vi "LowPressureVerification.vi"(8 "error in":errorcluster, 11 "S1 in":refnum<class "S4.lvclass">) -> (0 "error out":errorcluster, 3 "S1 out":refnum<class "S4.lvclass">)   [LabVIEW 2018, in "S4.lvclass"]
uses:
  S4.lvclass
  S4.lvclass/S4.ctl
  Public Controls/Outputs.ctl
  Public Controls/ReportHeader.ctl
  IO/IO.lvclass
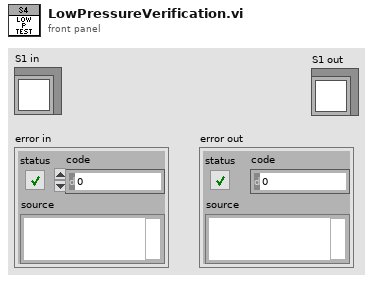
[diagram p1: front panel]
types:
  T1 = typedef "S4.lvclass/Outputs.ctl" = cluster{"LO P":bool, "HI P":bool, "Z3Vent":bool, "V2 Vent":bool, "IsLidLocked":bool}
  T2 = typedef "S4.lvclass/ReportHeader.ctl" = string
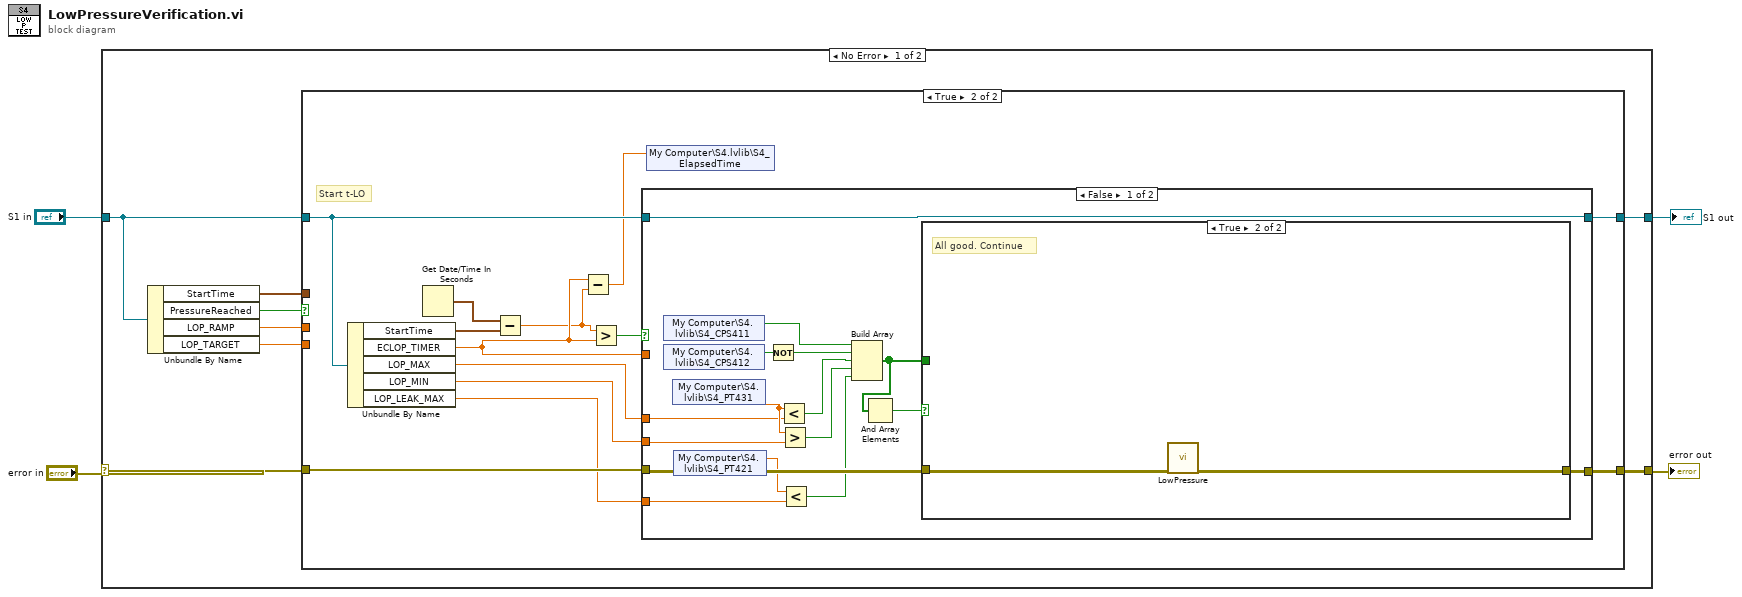
[diagram p0: block diagram]
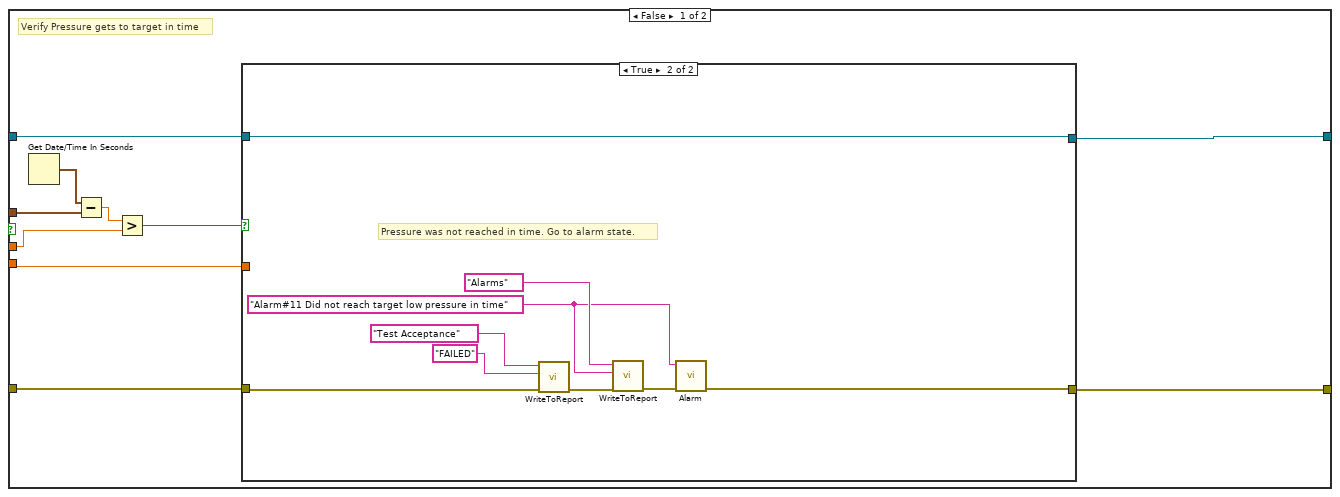
[diagram p2: hidden frame]
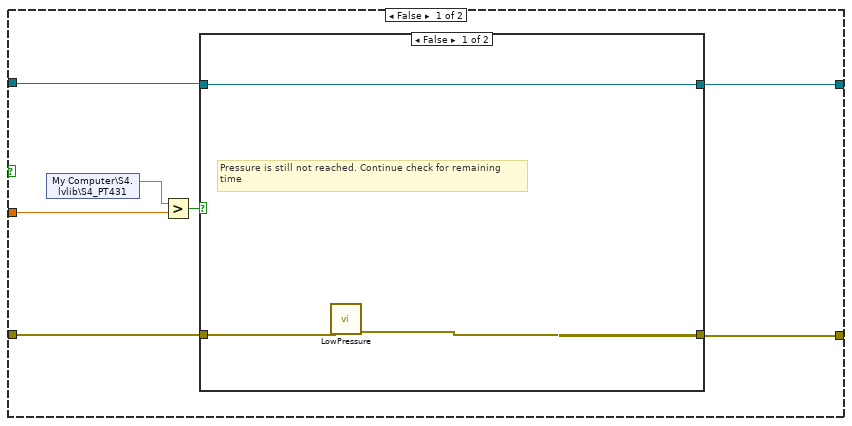
[diagram p3: hidden frame]
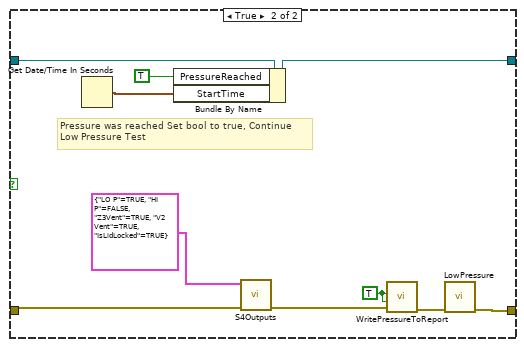
[diagram p4: hidden frame]
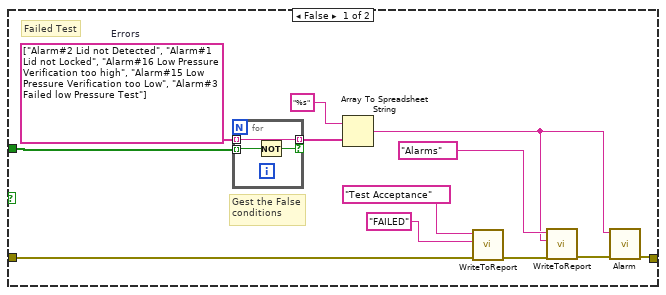
[diagram p5: hidden frame]
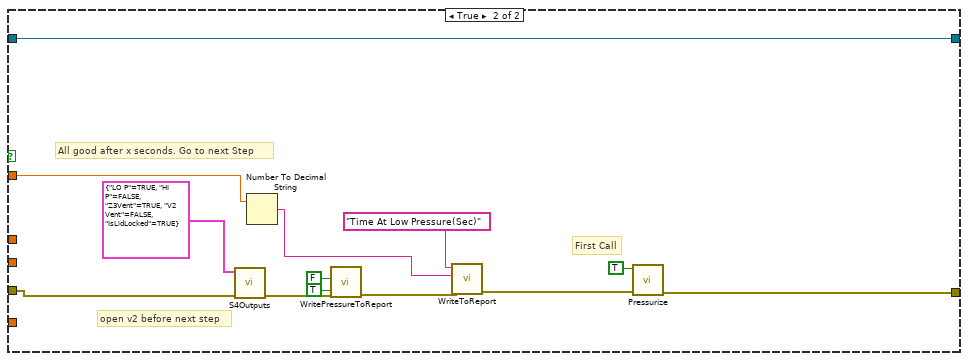
[diagram p6: hidden frame]
diagram:
  n1 = case shown="No Error" "error in" {
    selector: "error in" -> [w12 w113]
    tunnel: [w8 w113] -> w4
    tunnel: "S1 in" -> [w7 w112]
    tunnel: [w9 w112] -> w1
    frame No Error {
      n2 = Unbundle By Name(w7) -> ("StartTime"=w10:timestamp, "PressureReached"=w11:bool, "LOP_RAMP"=w6:dbl, "LOP_TARGET"=w5:dbl)
      n3 = case shown="True" w11 {
        tunnel: w12 -> [w19 w64]
        tunnel: [w17 w60] -> w8
        tunnel: w10 -> [w21 _]
        tunnel: w7 -> [w16 w59]
        tunnel: [w15 w58] -> w9
        tunnel: w6 -> [w14 _]
        tunnel: w5 -> [w13 _]
        frame False {
          # "Verify Pressure gets to target in time"
          n4 = Get Date/Time In Seconds() -> (seconds since 1Jan1904=w22:timestamp)
          n5 = Subtract(x=w22, y=w21) -> (x-y=w20:dbl)
          n6 = Greater?(x=w20, y=w14) -> (0:w18:bool)
          n7 = case shown="True" w18 {
            tunnel: w19 -> [w25 w46]
            tunnel: [w24 w48] -> w17
            tunnel: w16 -> [w27 w45]
            tunnel: [w26 w45] -> w15
            tunnel: w13 -> [w23 _]
            frame False {
              n8 = shared-variable "My Computer\\S4.lvlib\\S4_PT431"() -> (w29:dbl)  [unwired: 1 in, 1 out]
              n9 = Greater?(x=w29, y=w23) -> (0:w28:bool)
              n10 = case shown="False" w28 {
                tunnel: w27 -> [w31 w42]
                tunnel: [w31 w41] -> w26
                tunnel: w25 -> [w30 w34]
                tunnel: [w32 w36] -> w24
                frame False {
                  # "Pressure is still not reached. Continue check for remaining\ntime"
                  n11 = call "LowPressure.vi"("error in"=w30) -> ("error out"=w32:errorcluster)  [unwired: 10 in]
                }
                frame True {
                  w38 = TRUE ("Initial")
                  # "Pressure was reached Set bool to true, Continue\nLow Pressure Test"
                  n12 = Get Date/Time In Seconds() -> (seconds since 1Jan1904=w39:timestamp)
                  n13 = Bundle By Name(cluster=w42, "PressureReached"=TRUE ("PT111ReachedPressure"), "StartTime"=w39) -> (w41:refnum<class "S4.lvclass">)
                  n14 = call "S4Outputs.vi"("error in"=w34, "Outputs"=T1 {"LO P"=TRUE, "HI P"=FALSE, "Z3Vent"=TRUE, "V2 Vent"=TRUE, "IsLidLocked"=TRUE} ("SIOutputs")) -> ("error out"=w33:errorcluster)  [unwired: 9 in]
                  n15 = call "WritePressureToReport.vi"("error in (no error)"=w33, "LowPressure"=w38, "Initial"=w38) -> ("error out"=w37:errorcluster)  [unwired: 8 in]
                  n16 = call "LowPressure.vi"("error in"=w37) -> ("error out"=w36:errorcluster)  [unwired: 10 in]
                }
              }
            }
            frame True {
              w44 = "Alarm#11 Did not reach target low pressure in time" ("Value")
              # "Pressure was not reached in time. Go to alarm state."
              n17 = call "WriteToReport.vi"("error in"=w46, "Value"="FAILED", "Header"=T2 "Test Acceptance") -> ("error out"=w51:errorcluster)  [unwired: 8 in]
              n18 = call "WriteToReport.vi"("error in"=w51, "Value"=w44, "Header"="Alarms") -> ("error out"=w49:errorcluster)  [unwired: 8 in]
              n19 = call "Alarm.vi"("error in"=w49, "Alarm"=w44) -> ("error out"=w48:errorcluster)  [unwired: 9 in]
            }
          }
        }
        frame True {
          # "Start t-LO"
          n20 = Unbundle By Name(w59) -> ("StartTime"=w62:timestamp, "ECLOP_TIMER"=w57:dbl, "LOP_MAX"=w54:dbl, "LOP_MIN"=w53:dbl, "LOP_LEAK_MAX"=w52:dbl)
          n21 = Get Date/Time In Seconds() -> (seconds since 1Jan1904=w63:timestamp)
          n22 = Subtract(x=w63, y=w62) -> (x-y=w56:dbl)
          n23 = Subtract(x=w57, y=w56) -> (x-y=w55:dbl)
          n24 = Greater?(x=w56, y=w57) -> (0:w61:bool)
          n25 = case shown="False" w61 {
            tunnel: w64 -> [w81 w101]
            tunnel: [w78 w111] -> w60
            tunnel: w57 -> [_ w104]
            tunnel: w59 -> [w68 w102]
            tunnel: [w68 w102] -> w58
            tunnel: w54 -> [w67 _]
            tunnel: w53 -> [w66 _]
            tunnel: w52 -> [w65 _]
            frame False {
              n26 = shared-variable "My Computer\\S4.lvlib\\S4_CPS411"() -> (w72:bool)  [unwired: 1 in, 1 out]
              n27 = shared-variable "My Computer\\S4.lvlib\\S4_CPS412"() -> (w71:bool)  [unwired: 1 in, 1 out]
              n28 = shared-variable "My Computer\\S4.lvlib\\S4_PT431"() -> (w77:dbl)  [unwired: 1 in, 1 out]
              n29 = shared-variable "My Computer\\S4.lvlib\\S4_PT421"(error in=w81) -> (w80:dbl, error out=w79:errorcluster)
              n30 = Not(x=w71) -> (.not. x?=w69:bool)
              n31 = Less?(x=w77, y=w67) -> (x < y?=w76:bool)
              n32 = Greater?(x=w77, y=w66) -> (0:w75:bool)
              n33 = Less?(x=w80, y=w65) -> (x < y?=w70:bool)
              n34 = Build Array(w72, w69, w76, w75, w70) -> (w73:bool[])
              n35 = And Array Elements(Boolean array=w73) -> (logical AND=w74:bool)
              n36 = case shown="True" w74 {
                tunnel: w79 -> [w88 w98]
                tunnel: [w90 w97] -> w78
                tunnel: w73 -> [w87 _]
                frame False {
                  w86 = string[] ["Alarm#2 Lid not Detected", "Alarm#1 Lid not Locked", "Alarm#16 Low Pressure Verification too high", "Alarm#15 Low Pressure Verification too Low", "Alarm#3 Failed low Pressure Test"]  # Errors
                  # "Failed Test"
                  # "Gest the False\nconditions"
                  n37 = for {
                    tunnel: w87 -> [w95] mode=indexing
                    tunnel: w86 -> [w96] mode=indexing
                    tunnel: [w96] -> w85 mode=indexing if=w94
                    n38 = Not(x=w95) -> (.not. x?=w94:bool)
                  }
                  n39 = Array To Spreadsheet String(array=w85, 3:"%s" ("format string")) -> (spreadsheet string=w82:string)  [unwired: 1 in]
                  n40 = call "WriteToReport.vi"("error in"=w88, "Value"="FAILED", "Header"=T2 "Test Acceptance") -> ("error out"=w93:errorcluster)  [unwired: 8 in]
                  n41 = call "WriteToReport.vi"("error in"=w93, "Value"=w82, "Header"="Alarms") -> ("error out"=w91:errorcluster)  [unwired: 8 in]
                  n42 = call "Alarm.vi"("error in"=w91, "Alarm"=w82) -> ("error out"=w90:errorcluster)  [unwired: 9 in]
                }
                frame True {
                  # "All good. Continue"
                  n43 = call "LowPressure.vi"("error in"=w98) -> ("error out"=w97:errorcluster)  [unwired: 10 in]
                }
              }
            }
            frame True {
              # "open v2 before next step"
              # "First Call"
              # "All good after x seconds. Go to next Step"
              n44 = call "S4Outputs.vi"("error in"=w101, "Outputs"=T1 {"LO P"=TRUE, "HI P"=FALSE, "Z3Vent"=TRUE, "V2 Vent"=FALSE, "IsLidLocked"=TRUE} ("SIOutputs")) -> ("error out"=w99:errorcluster)  [unwired: 9 in]
              n45 = Number To Decimal String(number=w104) -> (decimal integer string=w103:string)  [unwired: 1 in]
              n46 = call "WritePressureToReport.vi"("error in (no error)"=w99, "LowPressure"=TRUE, "Initial"=FALSE) -> ("error out"=w107:errorcluster)  [unwired: 8 in]
              n47 = call "WriteToReport.vi"("error in"=w107, "Value"=w103, "Header"="Time At Low Pressure(Sec)") -> ("error out"=w106:errorcluster)  [unwired: 8 in]
              n48 = call "Pressurize.vi"("error in"=w106, "FirstCall(F)"=TRUE) -> ("error out"=w111:errorcluster)  [unwired: 9 in]
            }
          }
          n49 = shared-variable "My Computer\\S4.lvlib\\S4_ElapsedTime"(w55) -> ()  [unwired: 1 in, 1 out]
        }
      }
    }
    frame Error {
    }
  }
  "error out" <- w4
  "S1 out" <- w1
